vi "Get Debug Options.vi"(8 "error in":errorcluster, 11 "data sharing framework custom device in":T1 format="%.0x") -> (0 "error out":errorcluster, 1 "infinite FIFO timeouts?":bool, 2 "debug?":bool, 3 "data sharing framework custom device out":T1 format="%.0x")   [LabVIEW 2021, in "Data Sharing Framework Custom Device Scripting.lvlib"]
doc: "Reads the <b>debug?</b> and <b>infinite FIFO timeouts?</b> options. These options are available for all targets."
uses:
  Data Sharing Framework Custom Device Scripting.lvlib
  Shared/DSF Shared.lvlib
  <vilib>/NI VeriStand/Custom Device API/Custom Device Item Ref.ctl
  <vilib>/NI VeriStand/Custom Device API/Custom Device API.lvlib
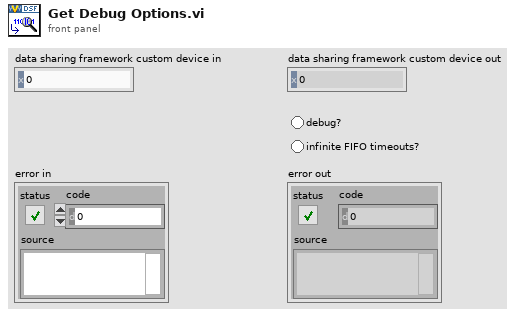
[diagram p1: front panel]
types:
  T1 = typedef "Custom Device API.lvlib/Custom Device Item Ref.ctl" = u64
  T2 = typedef "DSF Core.lvlibp/Framework.lvclass/Framework Options.ctl" = cluster{"FIFO Options":T3, "Thread Options":T4, "Plugin Options":T5, "Performance Options":T6, "Data Server Options":T7}
  T3 = typedef "DSF Core.lvlibp/Framework.lvclass/DSF FIFO Options.ctl" = cluster{"Infinite Timeouts":bool}
  T4 = typedef "DSF Core.lvlibp/Thread.lvclass/Thread Options.ctl" = cluster{"Show FP On Call":bool, "Close FP After Call":bool, "Allow Debugging":bool}
  T5 = typedef "DSF Core.lvlibp/Framework.lvclass/DSF Plugin Options.ctl" = cluster{"Default Components":bool}
  T6 = typedef "DSF Core.lvlibp/DSF Performance Options.ctl" = cluster{"Measure Period":bool, "Measure Rx/Tx Duration":bool}
  T7 = typedef "DSF Core.lvlibp/Framework.lvclass/Data Server Options.ctl" = cluster{"Enable Data Server":bool, "Period":u32}
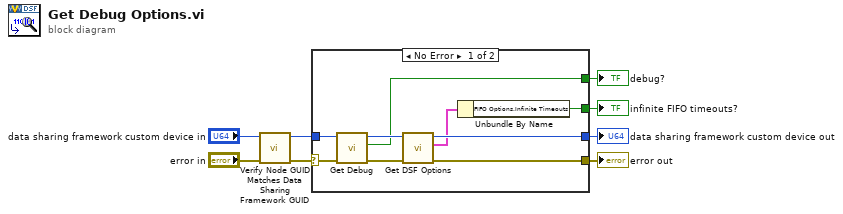
[diagram p0: block diagram]
diagram:
  n1 = call "Verify Node GUID Matches Data Sharing Framework GUID.vi"("error in"="error in", "data sharing framework custom device in"="data sharing framework custom device in") -> ("error out"=w1:errorcluster, "data sharing framework custom device out"=w2:T1)  [unwired: 8 in]
  n2 = case shown="No Error" w1 {
    selector: w1 -> [w9 w18]
    tunnel: [w17 w19] -> w8
    tunnel: [w16 w18] -> w7
    tunnel: [w14 _] -> w6
    tunnel: [w11 _] -> w5
    tunnel: w2 -> [w10 w19]
    frame No Error {
      n3 = call "Get Debug.vi"("error in (no error)"=w9, "Item Ref in"=w10) -> ("error out"=w13:errorcluster, "debug"=w11:bool, "Item Ref out"=w12:T1)  [unwired: 7 in]
      n4 = call "Get DSF Options.vi"("error in (no error)"=w13, "Item Ref in"=w12) -> ("error out"=w16:errorcluster, "options"=w15:T2, "Item Ref out"=w17:T1)  [unwired: 7 in]
      n5 = Unbundle By Name(w15) -> ("FIFO Options.Infinite Timeouts"=w14:bool)
    }
    frame Error {
    }
  }
  "data sharing framework custom device out" <- w8
  "error out" <- w7
  "infinite FIFO timeouts?" <- w6
  "debug?" <- w5
